vi "Error Handler.vi"(8 "error in (no error)":errorcluster, 9 "Is warning?":bool, 10 "Error message":string="Motic: unknown error", 11 "Function return":bool) -> (0 "error out":errorcluster)   [LabVIEW 2012, in "MoticApi.lvlib"]
uses:
  MoticApi.lvlib
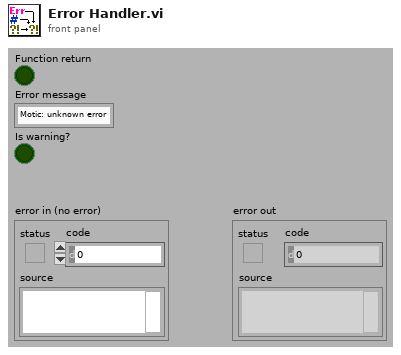
[diagram p1: front panel]
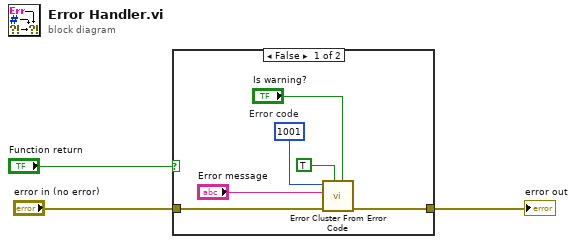
[diagram p0: block diagram]
diagram:
  n1 = case shown="False" "Function return" {
    tunnel: "error in (no error)" -> [w9 w10]
    tunnel: [w8 w10] -> w2
    frame False {
      w6 = 1001  # Error code
      n2 = call <vilib>:"Error Cluster From Error Code.vi"("is warning? (False)"="Is warning?", "show call chain? (False)"=TRUE, "error in (no error)"=w9, "error message (\"\")"="Error message", "error code (0)"=w6) -> ("error out"=w8:errorcluster)  [unwired: 4 in]
    }
    frame True {
    }
  }
  "error out" <- w2
